vi "HART_Read response.vi"(8 "error in":errorcluster, 10 "Max listen time\n(1000 ms)":u32=1000, 11 "resource name":refnum<visa-resource-name>) -> (0 "error out":errorcluster, 1 "unsigned byte array":u8[](array[numeric]) format="%.0x", 2 "Status (2 bytes)":u8[](array[numeric]) format="%.0x", 3 "Data bytes":u8[](array[numeric]) format="%.0x", 5 "Respons on\nCommand":u8 format="%.0x", 7 "Device Address (5 bytes)":u8[](array[numeric]) format="%.0x")   [LabVIEW 2016]
panel:
  out "Number read":u32
  out "string read":string
  # "1.....2........3.......4........5"
  # "86"
  # "/\\\n |"
  # "/\\\n |\n |\n |"
  # "address"
  # "8A3F115649"
  # "command"
  # "Bytecount (# of bytes to follow)"
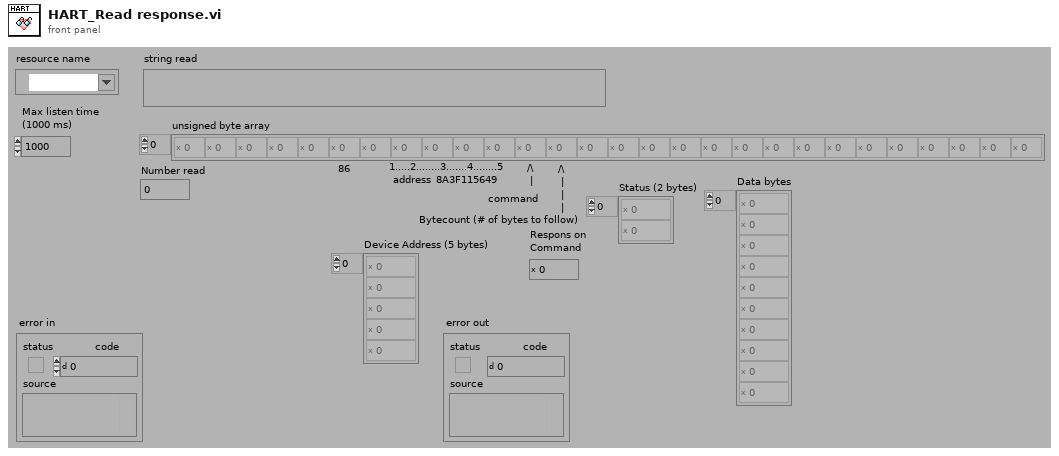
[diagram p1: front panel]
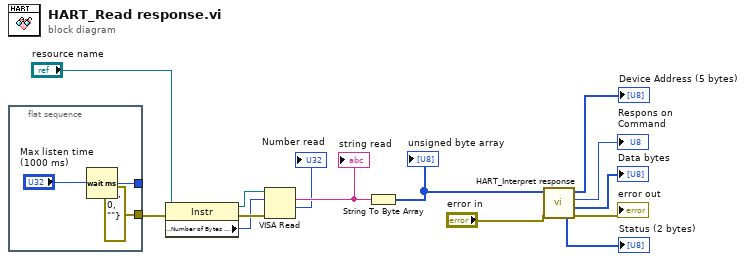
[diagram p0: block diagram]
diagram:
  n1 = flat-sequence {
    tunnel: [errorcluster {"status"=FALSE, "code"=0, "source"=""} ("error in")] -> w4
    tunnel: [w16] -> _
    frame #0 {
      n2 = Wait (ms)(milliseconds to wait="Max listen time\n(1000 ms)") -> (millisecond timer value=w16:u32)
    }
  }
  n3 = property class="Instr"(reference="resource name", error in=w4) -> (reference out=w1:refnum<visa-resource-name>, error out=w6:errorcluster, "Serial Settings:Number of Bytes at Serial Port"=w5:u32)
  n4 = VISA Read(VISA resource name=w1, byte count=w5, error in (no error)=w6) -> (read buffer=w7:string, return count=→"Number read":u32)  [unwired: 2 out]
  "string read" <- w7
  n5 = String To Byte Array(string=w7) -> (unsigned byte array=w14:u8[])
  "unsigned byte array" <- w14
  n6 = call "HART_Interpret response.vi"("error in"="error in", "byte array"=w14) -> ("error out"=→"error out":errorcluster, "Data bytes"=→"Data bytes":u8[], "Respons on\nCommand"=→"Respons on\nCommand":u8, "Device Address\n(5 bytes)"=→"Device Address (5 bytes)":u8[], "Status (2 bytes)"=→"Status (2 bytes)":u8[])  [unwired: 5 in]
